vi "ADQ214 GetAcquiredAll (ILYA).vi"(8 "error in":errorcluster, 11 "adq_cu_ptr":u32) -> (0 "error out":errorcluster, 2 "return":u32, 3 "adq_cu_ptr":u32)   [LabVIEW 2013]
uses:
  dlls/ADQAPI.dll
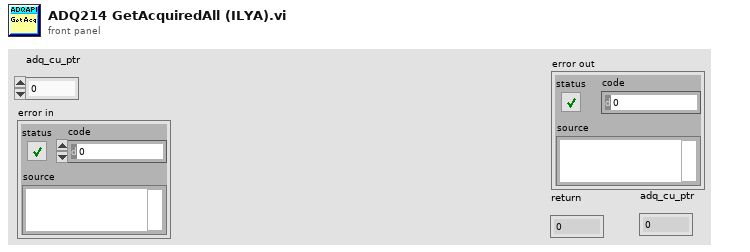
[diagram p1: front panel]
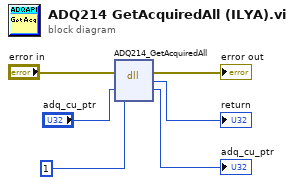
[diagram p0: block diagram]
diagram:
  n1 = dll-call lib="C:/Users/astafiev/Desktop/IlyaDrive/@photonCounting/LabView_Imperium/dlls/ADQAPI.dll" fn="ADQ214_GetAcquiredAll"(error in="error in", "adq_cu_ptr"="adq_cu_ptr", "adq_num"=1) -> (error out=→"error out":errorcluster, "return type"=→"return":u32, "adq_cu_ptr"=→"adq_cu_ptr":u32)  [unwired: 3 in, 1 out]
